vi "UTIL_CalibratePropmt.vi"(11 "Sequence":i32) -> (3 "Input Out":string)   [LabVIEW 2024]
panel:
  in  "OK Button":bool
  in  "INPUT":string
  out "CALIBRATION":string="START LEVEL CALIBRATION:\n1.  Set the pump to a Empty level.\n2.  Press \"OK\" when ready to measure."
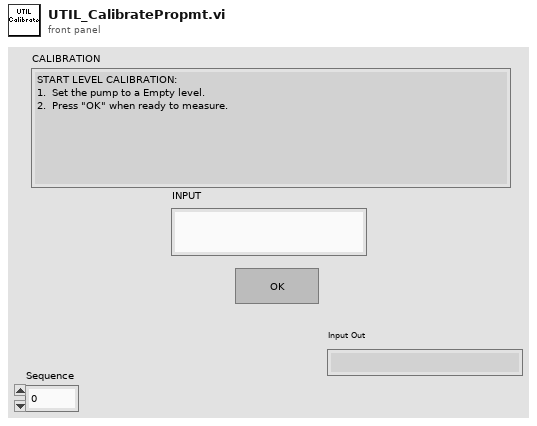
[diagram p1: front panel]
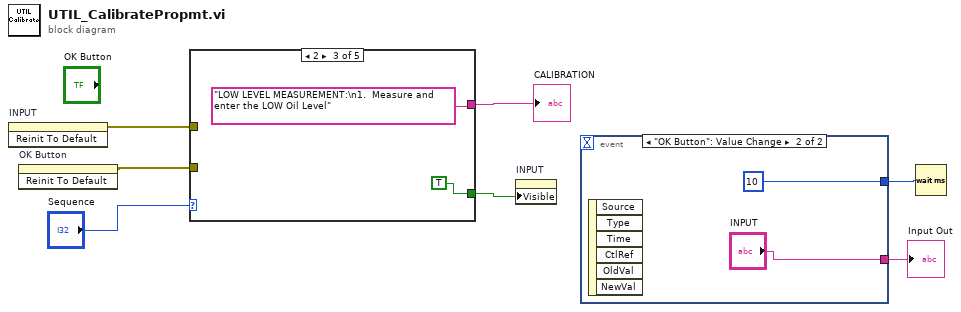
[diagram p0: block diagram]
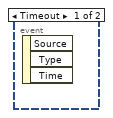
[diagram p2: hidden frame]
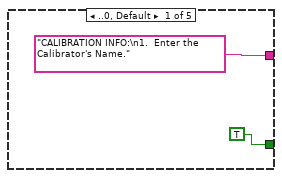
[diagram p3: hidden frame]
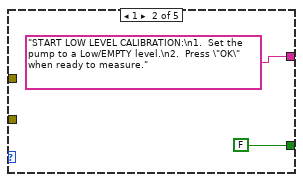
[diagram p4: hidden frame]
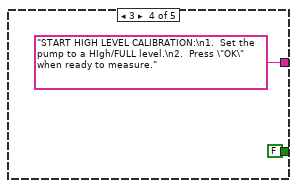
[diagram p5: hidden frame]
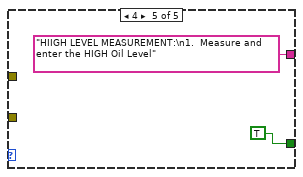
[diagram p6: hidden frame]
diagram:
  n1 = invoke on="INPUT" class="Str" method="Reinit To Default"() -> (error out=w7:errorcluster)  [unwired: 3 in, 2 out]
  n2 = invoke on="OK Button" class="Bool (strict)" method="Reinit To Default"() -> (error out=w6:errorcluster)  [unwired: 3 in, 2 out]
  n3 = case shown="2" "Sequence" {
    tunnel: w7 -> [_ _ _ _ _]
    tunnel: w6 -> [_ _ _ _ _]
    tunnel: ["CALIBRATION INFO:\n1.  Enter the Calibrator's Name." "START LOW LEVEL CALIBRATION:\n1.  Set the pump to a Low/EMPTY level.\n2.  Press \"OK\" when ready to measure." "LOW LEVEL MEASUREMENT:\n1.  Measure and enter the LOW Oil Level" "START HIGH LEVEL CALIBRATION:\n1.  Set the pump to a HIgh/FULL level.\n2.  Press \"OK\" when ready to measure." "HIIGH LEVEL MEASUREMENT:\n1.  Measure and enter the HIGH Oil Level"] -> w4
    tunnel: [TRUE FALSE ("Boolean") TRUE FALSE TRUE] -> w3
    frame ..0, Default {
    }
    frame 1 {
    }
    frame 2 {
    }
    frame 3 {
    }
    frame 4 {
    }
  }
  "CALIBRATION" <- w4
  n4 = property on="INPUT" class="Str"("Visible"=w3) -> ()  [unwired: 2 in, 2 out]
  n5 = event shown="[1] \"OK Button\": Value Change" {
    selector: _ -> [_ _]
    dyn-events: _ -> [_ _]
    timeout: _ -> [_ _]
    tunnel: [_ "INPUT"] -> w2
    tunnel: [_ u32 10 ("milliseconds to wait")] -> w1
    event Timeout {
      n6 = event-data() -> ()  [unwired: 1 in, 3 out]
    }
    event "OK Button": Value Change {
      n7 = event-data() -> ()  [unwired: 1 in, 6 out]
    }
  }
  "Input Out" <- w2
  n8 = Wait (ms)(milliseconds to wait=w1) -> ()  [unwired: 1 out]
